vi "testNoError.vi"() -> (0 "error out":errorcluster)   [LabVIEW 2019, in "TestCaseTest.lvlib" / "Fact.lvlib"]
uses:
  Fact.lvlib
  TestCase/Fact/Fact.lvclass
  Assertion/Assertion.lvlib
  TestCaseTestSupport/TestCaseTestSupport.lvlib
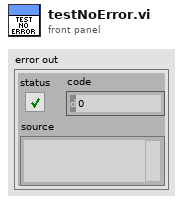
[diagram p1: front panel]
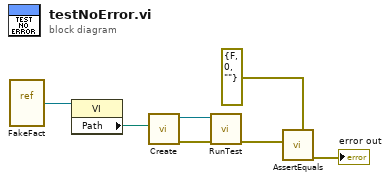
[diagram p0: block diagram]
diagram:
  n1 = vi-ref "FakeFact.vi"() -> (w3:refnum<vi>)
  n2 = property class="VI"(reference=w3) -> ("Path"=w2:path)  [unwired: 1 in, 2 out]
  n3 = call "Create.vi"("Path"=w2) -> ("error out"=w6:errorcluster, "Fact"=w7:refnum<class "Fact.lvclass">)  [unwired: 9 in]
  n4 = call-dynamic "RunTest.vi"("error in (no error)"=w6, "Fact in"=w7) -> ("error out"=w5:errorcluster)  [unwired: 8 in, 1 out]
  n5 = call "AssertEquals.vi"("Expected"=errorcluster {"status"=FALSE, "code"=0, "source"=""} ("error out"), "Actual"=w5) -> ("error out"=→"error out":errorcluster)  [unwired: 9 in]
